vi "5700C Wrapper.vi"(6 "Measurement Type":i32(ring)=1 items=["Current", "Voltage", "Power"], 7 "States":T2=enum."Config", 8 "error in":errorcluster, 9 "Enable Output":bool=TRUE, 10 "Setting":T1={"Max Volt"=10.0, "Voltage Set"=5.0, "Current Lim"=0.5}, 11 "Alias":string="PS4") -> (0 "error out":errorcluster, 1 "Over Current?":bool caption="in state", 2 "Over Voltage?":bool caption="in state", 3 "Measurement":dbl=nan)   [LabVIEW 2021]
doc: "This is a wrapper to support Keysight N6700C."
uses:
  Load INI/Controls/PowerSupply_Data.ctl
  Controls/PS States.ctl
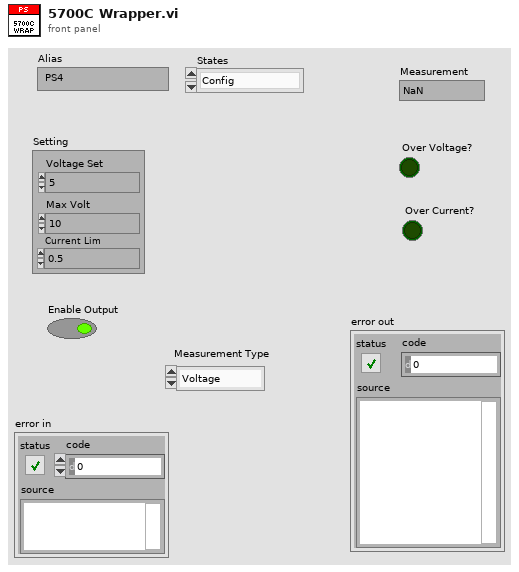
[diagram p1: front panel]
types:
  T1 = cluster{"Max Volt":dbl, "Voltage Set":dbl, "Current Lim":dbl}
  T2 = typedef "PS States.ctl" = enum16{"Init", "Config", "Enable Output", "Measure", "Close"}
  T3 = typedef "PowerSupply_Data.ctl" = cluster{"Alias":string, "Device":string, "Channel name":string}
  T4 = cluster{"Channel Name":string, "instrument handle":refnum<k15>}
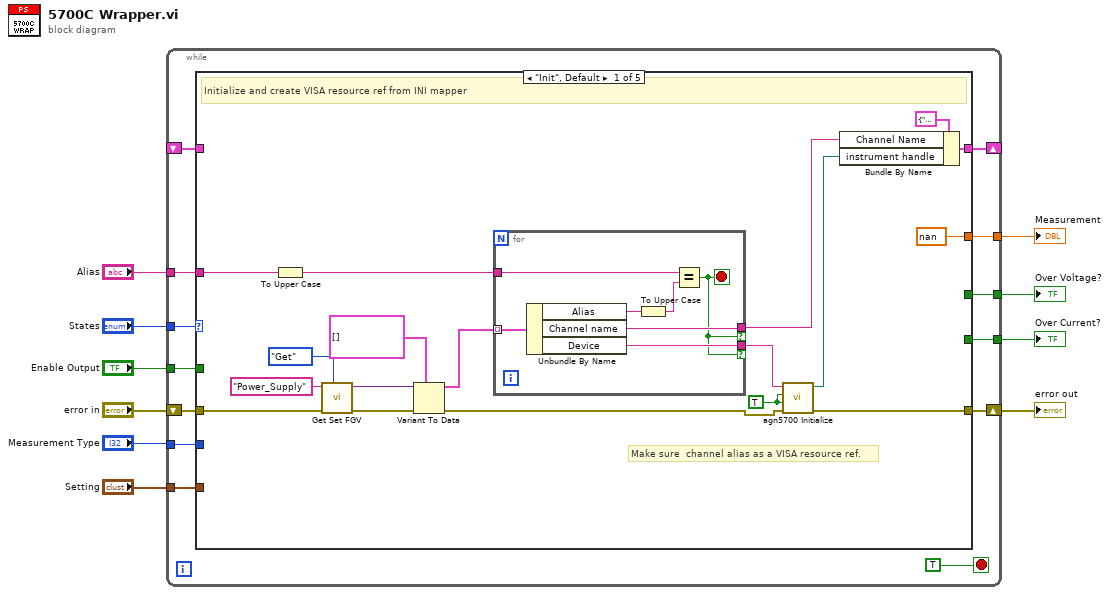
[diagram p0: block diagram]
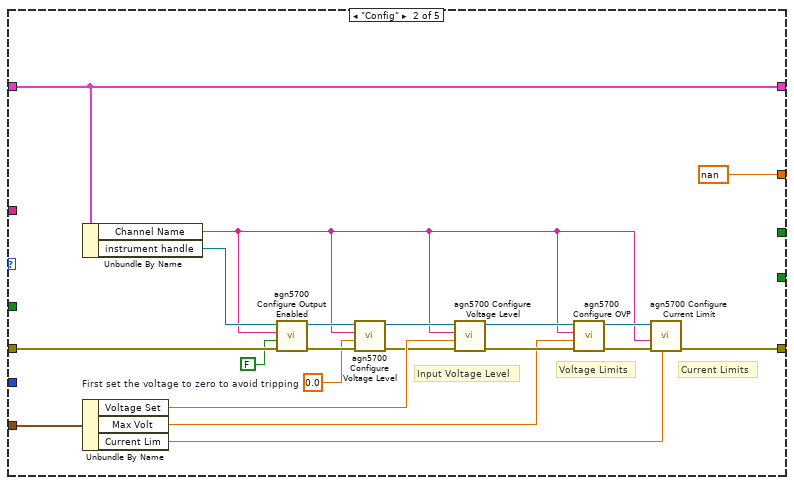
[diagram p2: hidden frame]
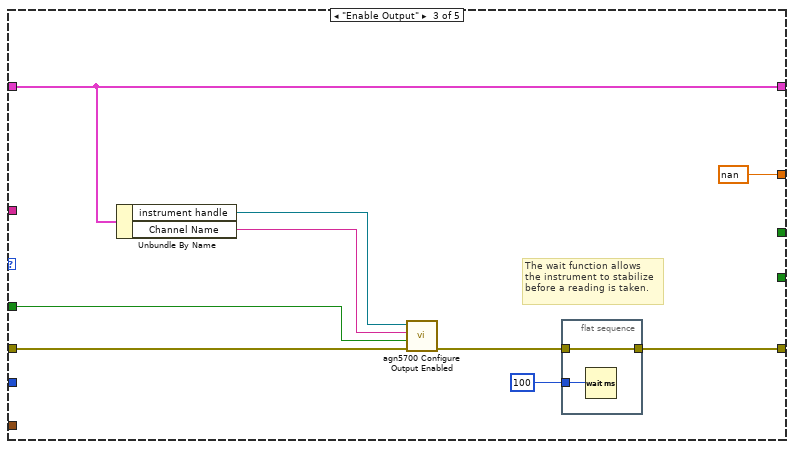
[diagram p3: hidden frame]
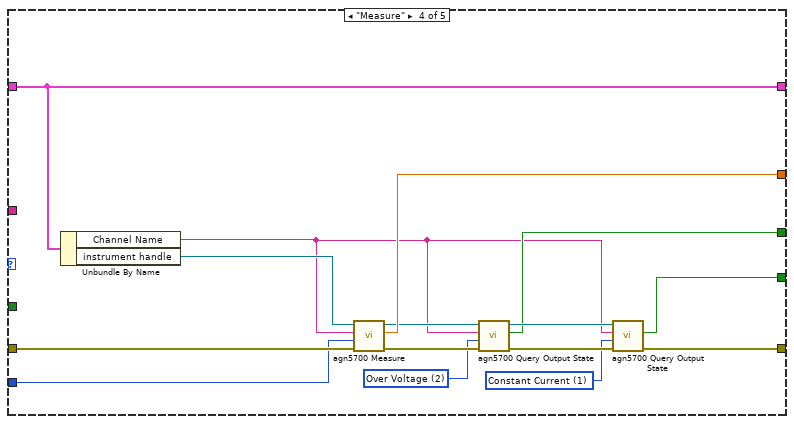
[diagram p4: hidden frame]
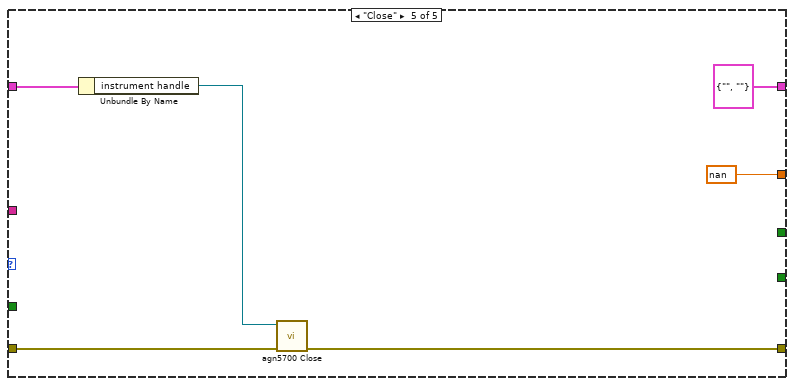
[diagram p5: hidden frame]
diagram:
  n1 = while {
    tunnel: "States" -> [w22]
    tunnel: "Enable Output" -> [w18]
    tunnel: "Setting" -> [w17]
    tunnel: [w15] -> w4
    shift-right: [w21] -> w8
    shift-left: "error in" -> [w23]
    shift-right: [w20] -> _
    shift-left: _ -> [w19]
    tunnel: "Alias" -> [w16]
    tunnel: "Measurement Type" -> [w14]
    tunnel: [w12] -> w2
    tunnel: [w11] -> w1
    stop <- TRUE stop-if-true
    n2 = case shown="\"Init\", Default" w22 {
      tunnel: w23 -> [w39 w54 w73 w92 w97]
      tunnel: [w26 w58 w76 w85 w95] -> w21
      tunnel: [w40 w68 w77 w94 T4 {"Channel Name"="", "instrument handle"=""}] -> w20
      tunnel: w19 -> [_ w68 w77 w94 w100]
      tunnel: [nan nan nan w91 nan] -> w15
      tunnel: w18 -> [_ _ w69 _ _]
      tunnel: w17 -> [_ w67 _ _ _]
      tunnel: w16 -> [w33 _ _ _ _]
      tunnel: w14 -> [_ _ _ w90 _]
      tunnel: [_ _ _ w83 _] -> w12
      tunnel: [_ _ _ w80 _] -> w11
      frame "Init", Default {
        w28 = TRUE ("reset device (true)")
        # "Make sure  channel alias as a VISA resource ref."
        # "Initialize and create VISA resource ref from INI mapper"
        n3 = To Upper Case(1:w33) -> (0:w32:string)
        n4 = call "Get Set FGV.vi"("Method (Get)"=enum16{"Get", "Set"}."Get", "error in"=w39, "Name"="Power_Supply") -> ("error out"=w37:errorcluster, "Data out"=w36:variant)  [unwired: 7 in]
        n5 = Variant To Data(error in=w37, type=T3[] [], Variant=w36) -> (data=w34:T3[], error out=w27:errorcluster)
        n6 = for {
          tunnel: w34 -> [w48] mode=indexing
          tunnel: w32 -> [w47]
          tunnel: [w44] -> w25 if=w42
          tunnel: [w43] -> w31 if=w42
          stop <- w42 stop-if-true
          n7 = Unbundle By Name(w48) -> ("Alias"=w45:string, "Channel name"=w43:string, "Device"=w44:string)
          n8 = To Upper Case(1:w45) -> (0:w46:string)
          n9 = Equal?(x=w47, y=w46) -> (x = y?=w42:bool)
        }
        n10 = call <instrlib>:"agn5700 Initialize.vi"("error in (no error)"=w27, "reset device (Yes)"=w28, "id query (Yes)"=w28, "resource name"=w25) -> ("error out"=w26:errorcluster, "instrument handle out"=w24:refnum<k15>)  [unwired: 6 out]
        n11 = Bundle By Name(cluster=T4 {"Channel Name"="", "instrument handle"=""}, "Channel Name"=w31, "instrument handle"=w24) -> (w40:T4)
      }
      frame "Config" {
        w56 = 0.0  # First set the voltage to zero to avoid tripping
        # "Current Limits"
        # "Voltage Limits"
        # "Input Voltage Level"
        n12 = Unbundle By Name(w68) -> ("Channel Name"=w50:string, "instrument handle"=w53:refnum<k15>)
        n13 = Unbundle By Name(w67) -> ("Voltage Set"=w61:dbl, "Max Volt"=w60:dbl, "Current Lim"=w59:dbl)
        n14 = call <instrlib>:"agn5700 Configure Output Enabled.vi"("error in (no error)"=w54, "enabled (True)"=FALSE, "channel name (\"\")"=w50, "instrument handle"=w53) -> ("error out"=w57:errorcluster, "instrument handle out"=w52:refnum<k15>)  [unwired: 6 out]
        n15 = call <instrlib>:"agn5700 Configure Voltage Level.vi"("error in (no error)"=w57, "level (0.02)"=w56, "channel name (\"\")"=w50, "instrument handle"=w52) -> ("error out"=w55:errorcluster, "instrument handle out"=w51:refnum<k15>)  [unwired: 6 out]
        n16 = call <instrlib>:"agn5700 Configure Voltage Level.vi"("error in (no error)"=w55, "level (0.02)"=w61, "channel name (\"\")"=w50, "instrument handle"=w51) -> ("error out"=w65:errorcluster, "instrument handle out"=w63:refnum<k15>)  [unwired: 6 out]
        n17 = call <instrlib>:"agn5700 Configure OVP.vi"("error in (no error)"=w65, "limit (5.0)"=w60, "channel name (\"\")"=w50, "instrument handle"=w63) -> ("error out"=w64:errorcluster, "instrument handle out"=w62:refnum<k15>)  [unwired: 1 in, 5 out]
        n18 = call <instrlib>:"agn5700 Configure Current Limit.vi"("limit (0.0)"=w59, "error in (no error)"=w64, "channel name (\"\")"=w50, "instrument handle"=w62) -> ("error out"=w58:errorcluster)  [unwired: 1 in, 6 out]
      }
      frame "Enable Output" {
        # "The wait function allows \nthe instrument to stabilize\nbefore a reading is taken."
        n19 = Unbundle By Name(w77) -> ("instrument handle"=w71:refnum<k15>, "Channel Name"=w70:string)
        n20 = call <instrlib>:"agn5700 Configure Output Enabled.vi"("error in (no error)"=w73, "enabled (True)"=w69, "channel name (\"\")"=w70, "instrument handle"=w71) -> ("error out"=w72:errorcluster)  [unwired: 7 out]
        n21 = flat-sequence {
          tunnel: [w79] -> w76
          tunnel: w72 -> [w79]
          tunnel: u32 100 ("milliseconds to wait") -> [w78]
          frame #0 {
            n22 = Wait (ms)(milliseconds to wait=w78) -> ()  [unwired: 1 out]
          }
        }
      }
      frame "Measure" {
        w81 = 1 items=["Constant Voltage"=0, "Constant Current"=1, "Unregulated"=4, "Over Voltage"=2, "Over Current"=3, "Over temperature"=1001, "Wait transient trigger"=1002, "Inhibit signals"=1003, "Power failed"=1004] ("output state (Constant Voltage)")
        w87 = 2 items=["Constant Voltage"=0, "Constant Current"=1, "Unregulated"=4, "Over Voltage"=2, "Over Current"=3, "Over temperature"=1001, "Wait transient trigger"=1002, "Inhibit signals"=1003, "Power failed"=1004] ("output state (Constant Voltage)")
        n23 = Unbundle By Name(w94) -> ("Channel Name"=w82:string, "instrument handle"=w93:refnum<k15>)
        n24 = call <instrlib>:"agn5700 Measure.vi"("error in (no error)"=w92, "measurement type (Voltage)"=w90, "channel name (\"\")"=w82, "instrument handle"=w93) -> ("error out"=w88:errorcluster, "measurement"=w91:dbl, "instrument handle out"=w89:refnum<k15>)  [unwired: 5 out]
        n25 = call <instrlib>:"agn5700 Query Output State.vi"("error in (no error)"=w88, "output state (Constant Voltage)"=w87, "channel name (\"\")"=w82, "instrument handle"=w89) -> ("error out"=w86:errorcluster, "in state"=w83:bool, "instrument handle out"=w84:refnum<k15>)  [unwired: 5 out]
        n26 = call <instrlib>:"agn5700 Query Output State.vi"("error in (no error)"=w86, "output state (Constant Voltage)"=w81, "channel name (\"\")"=w82, "instrument handle"=w84) -> ("error out"=w85:errorcluster, "in state"=w80:bool)  [unwired: 6 out]
      }
      frame "Close" {
        n27 = Unbundle By Name(w100) -> ("instrument handle"=w96:refnum<k15>)
        n28 = call <instrlib>:"agn5700 Close.vi"("error in (no error)"=w97, "instrument handle"=w96) -> ("error out"=w95:errorcluster)  [unwired: 9 out]
      }
    }
  }
  "error out" <- w8
  "Measurement" <- w4
  "Over Voltage?" <- w2
  "Over Current?" <- w1
